vi "Configure Channel.vi"(0 "VISA resource name":refnum<visa-resource-name>, 1 "Enable Channel (T: Enable)":bool=TRUE, 2 "Input Impedance (0: 1M ohm)":u16(ring) items=["1M", "50"], 3 "Bandwidth (0: FULL)":u16(ring) items=["FULL", "500 MHz", "250 MHz", "150 MHz", "20 MHz"], 5 "Channel (0: Channel 1)":u16(ring) format="%#_5f" items=["Channel 1", "Channel 2", "Channel 3", "Channel 4", "Math 1", "Math 2", "Math 3", "Math 4", "Reference 1", "Reference 2", "Reference 3", "Reference 4"], 7 "Vertical Coupling (1: DC)":u16(ring)=1 items=["AC", "DC", "Ground"], 9 "Probe Attenuation (1.0)":dbl=1.0, 11 "error in (no error)":errorcluster, 12 "Vertical Range (10.0 V)":dbl=10.0, 13 "Vertical Offset (0.0 V)":dbl) -> (4 "VISA resource name out":refnum<visa-resource-name>, 15 "error out":errorcluster)   [LabVIEW 2011, in "Tektronix 7000 Series.lvlib"]
doc: "Configures the vertical properties of an oscilloscope for a specified channel. This VI does not configure channel settings for disabled channels."
uses:
  Tektronix 7000 Series.lvlib
panel:
  # "Input Channel Parameters"
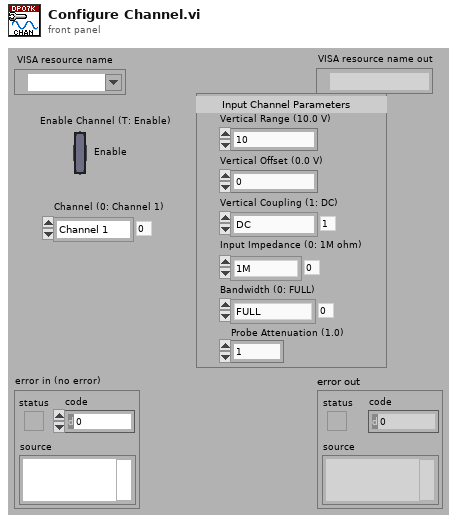
[diagram p1: front panel]
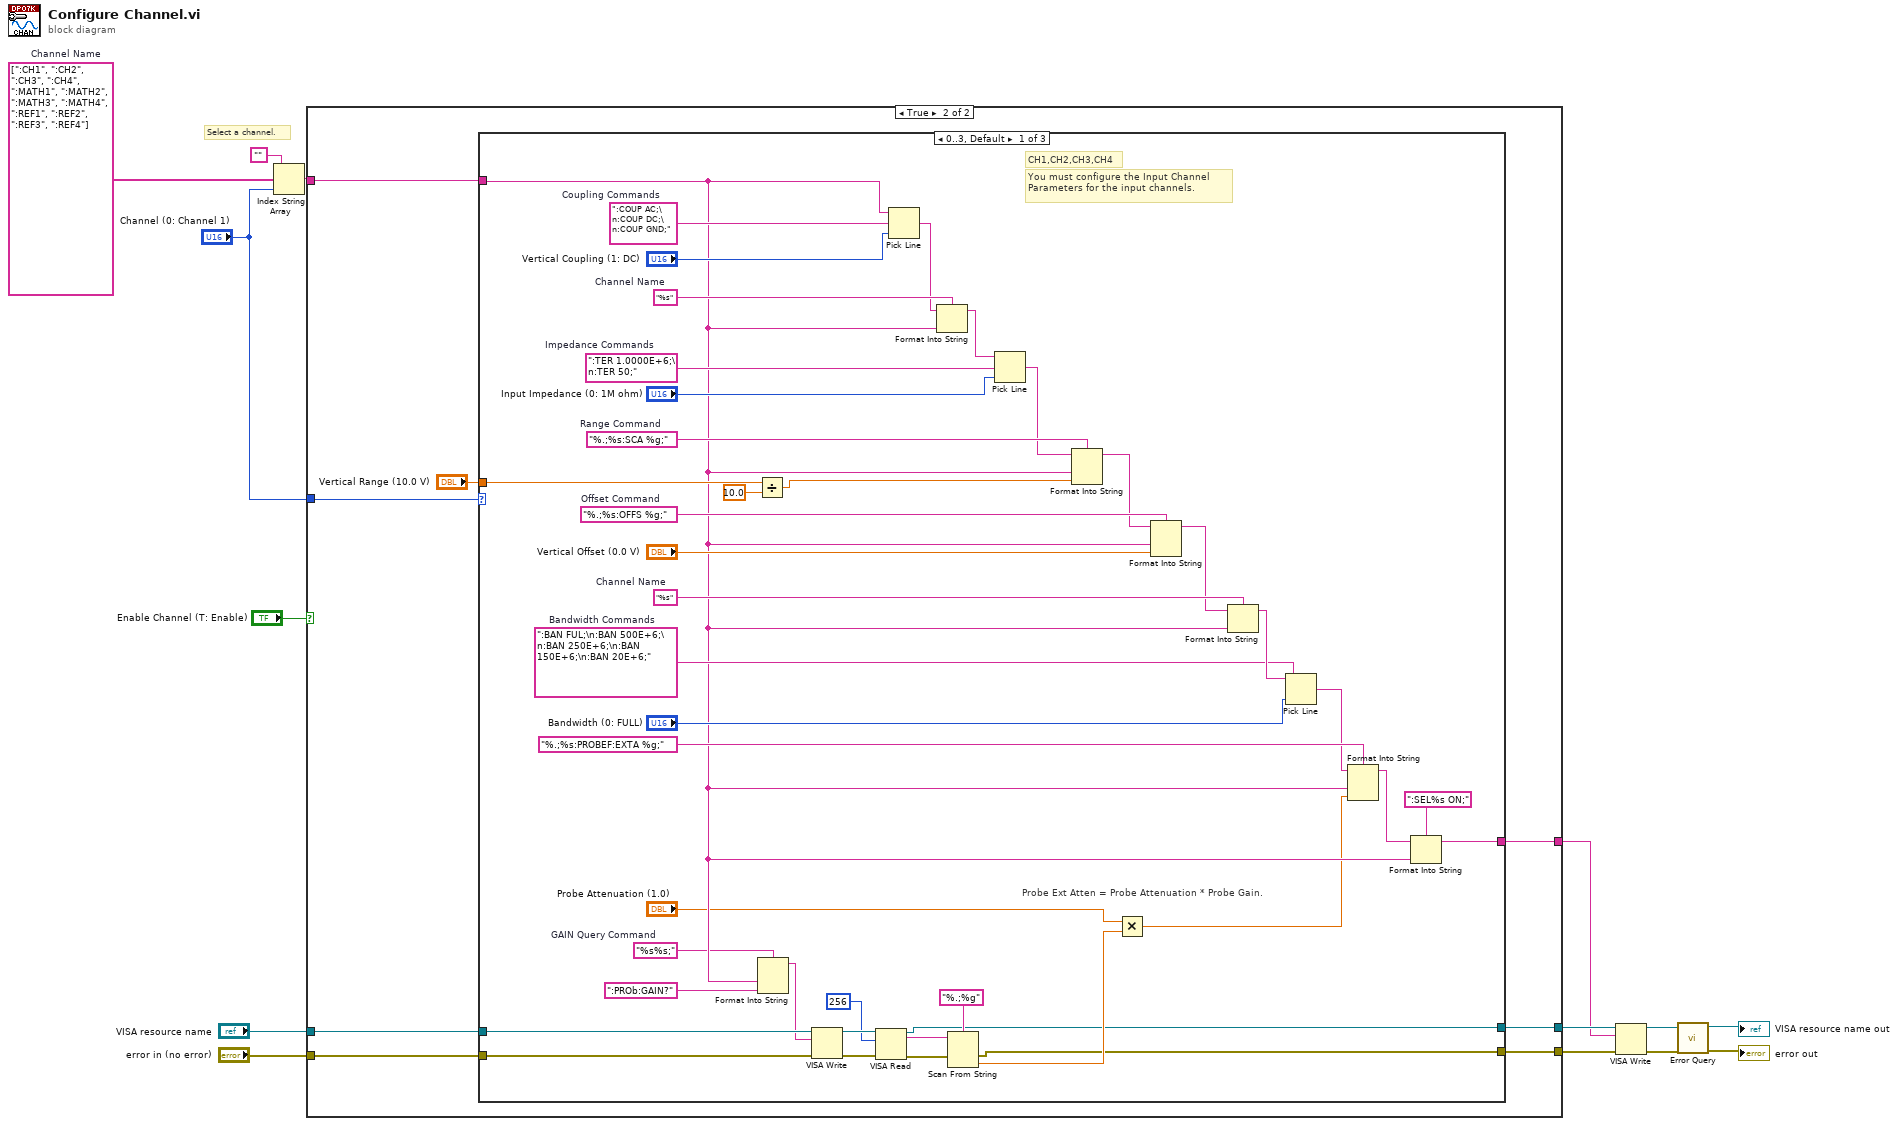
[diagram p0: block diagram]
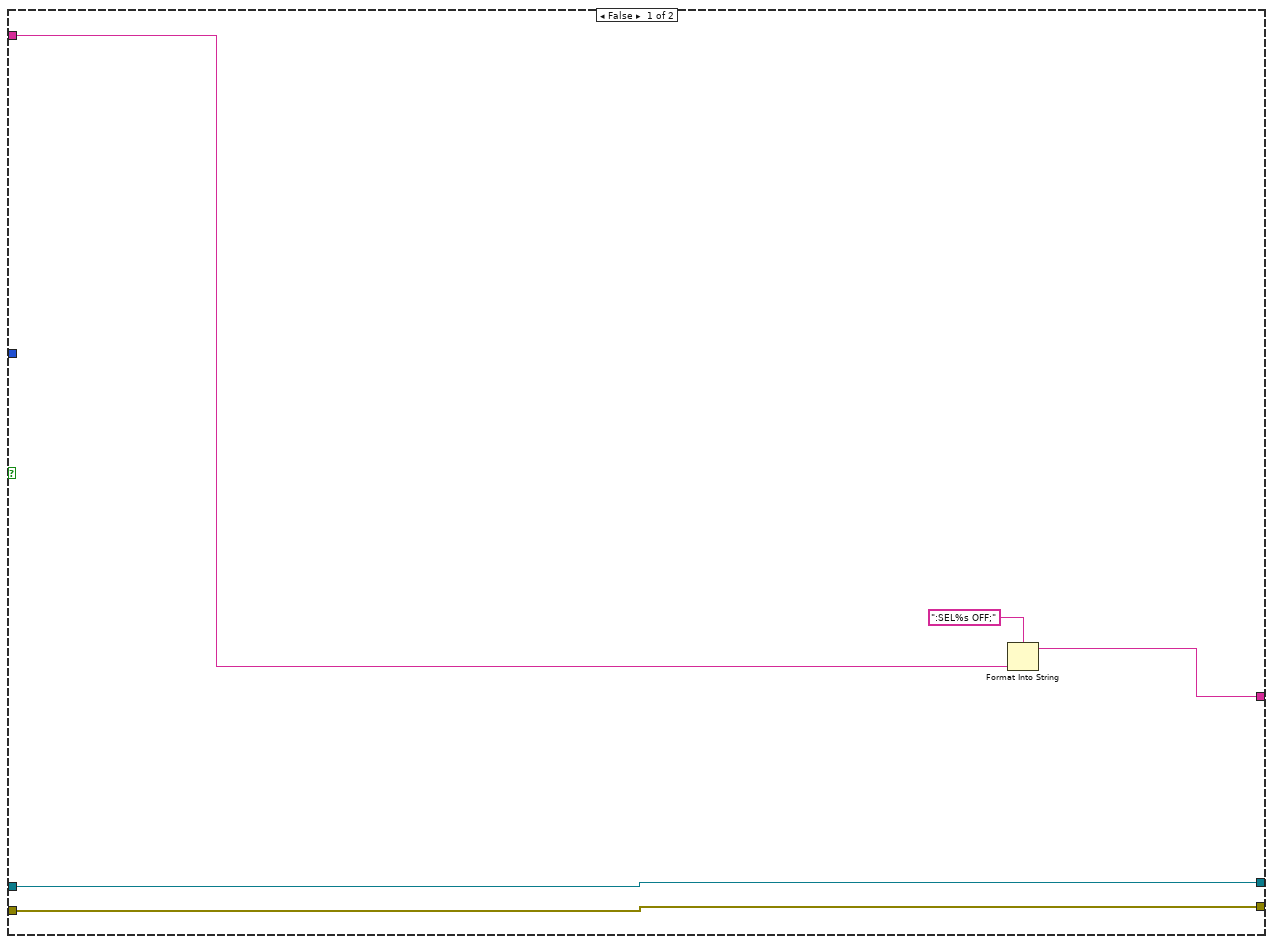
[diagram p2: hidden frame]
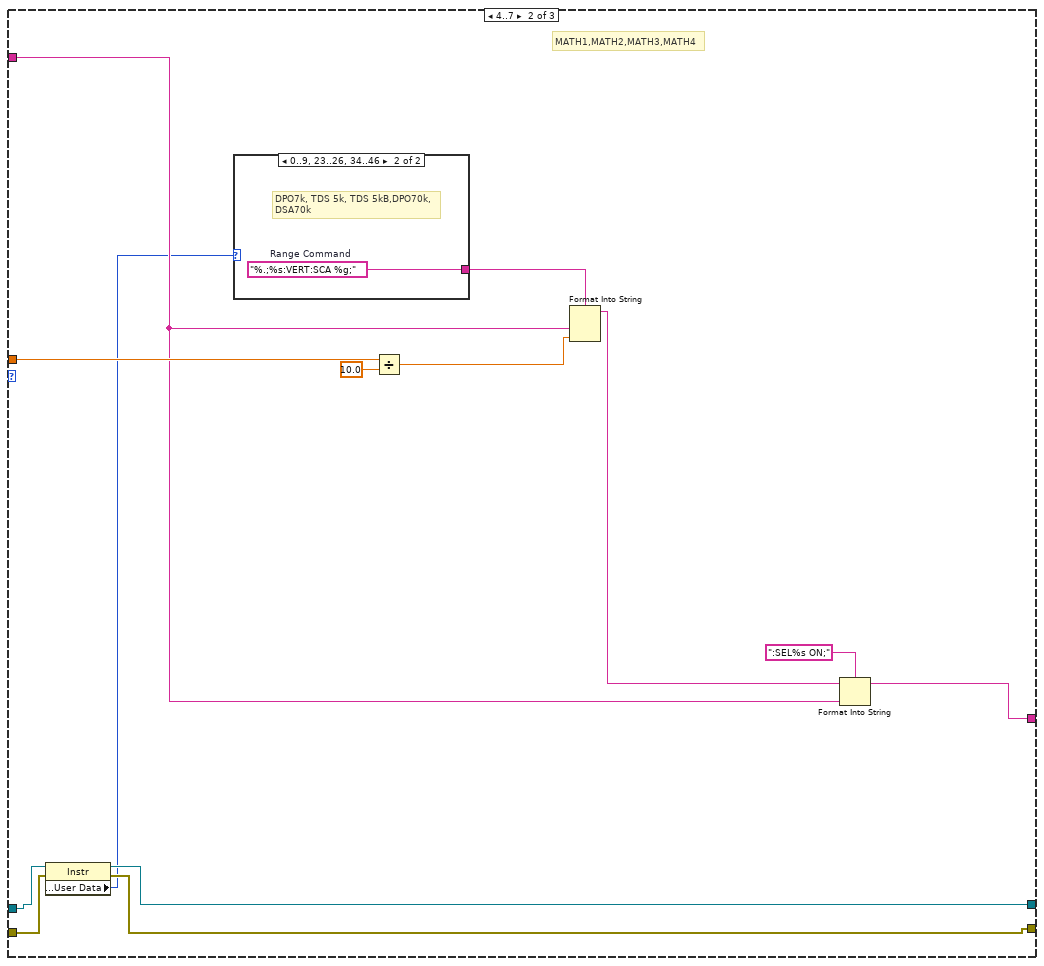
[diagram p3: hidden frame]
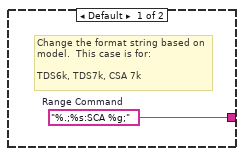
[diagram p4: hidden frame]
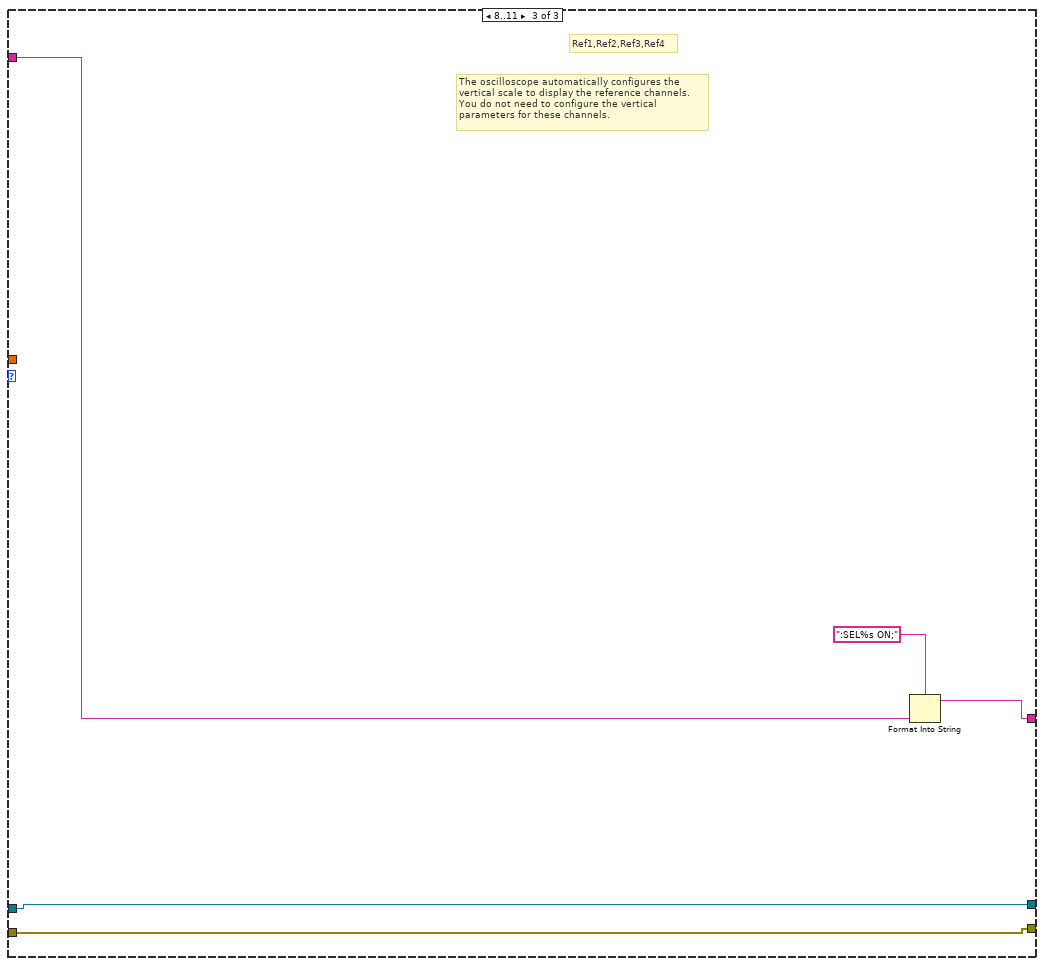
[diagram p5: hidden frame]
diagram:
  w11 = string[] [":CH1", ":CH2", ":CH3", ":CH4", ":MATH1", ":MATH2", ":MATH3", ":MATH4", ":REF1", ":REF2", ":REF3", ":REF4"]  # Channel Name
  # "Select a channel."
  n1 = Index String Array(1:"Channel (0: Channel 1)", 2:w11, 3:"" ("Empty String Constant")) -> (0:w12:string)
  n2 = case shown="True" "Enable Channel (T: Enable)" {
    tunnel: w12 -> [w19 w27]
    tunnel: "Channel (0: Channel 1)" -> [_ w26]
    tunnel: "VISA resource name" -> [w16 w24]
    tunnel: "error in (no error)" -> [w15 w23]
    tunnel: [w16 w22] -> w3
    tunnel: [w15 w21] -> w2
    tunnel: [w17 w20] -> w1
    frame False {
      n3 = Format Into String(format string=":SEL%s OFF;", w19) -> (resulting string=w17:string)  [unwired: 2 in, 1 out]
    }
    frame True {
      n4 = case shown="0..3, Default" w26 {
        tunnel: w27 -> [w42 w77 w88]
        tunnel: "Vertical Range (10.0 V)" -> [w57 w80 _]
        tunnel: w24 -> [w45 w74 w86]
        tunnel: w23 -> [w44 w73 w85]
        tunnel: [w30 w72 w86] -> w22
        tunnel: [w29 w71 w85] -> w21
        tunnel: [w28 w76 w87] -> w20
        frame 0..3, Default {
          w41 = "%s%s;"  # GAIN Query Command
          w48 = "%.;%s:OFFS %g;"  # Offset Command
          w53 = "%s"  # Channel Name
          w54 = ":TER 1.0000E+6;\n:TER 50;"  # Impedance Commands
          w56 = "%.;%s:SCA %g;"  # Range Command
          w65 = ":BAN FUL;\n:BAN 500E+6;\n:BAN 250E+6;\n:BAN 150E+6;\n:BAN 20E+6;"  # Bandwidth Commands
          w67 = "%s"  # Channel Name
          w69 = ":COUP AC;\n:COUP DC;\n:COUP GND;"  # Coupling Commands
          # "CH1,CH2,CH3,CH4"
          # "Probe Ext Atten = Probe Attenuation * Probe Gain."
          # "You must configure the Input Channel\nParameters for the input channels."
          n5 = Divide(x=w57, y=10.0) -> (x/y=w61:dbl)
          n6 = Format Into String(format string=w41, w42, ":PROb:GAIN?" ("write buffer")) -> (resulting string=w40:string)  [unwired: 2 in, 1 out]
          n7 = VISA Write(VISA resource name=w45, write buffer=w40, error in (no error)=w44) -> (VISA resource name out=w39:refnum<visa-resource-name>, error out=w38:errorcluster)  [unwired: 1 out]
          n8 = VISA Read(VISA resource name=w39, byte count=u32 256, error in (no error)=w38) -> (VISA resource name out=w30:refnum<visa-resource-name>, read buffer=w35:string, error out=w36:errorcluster)  [unwired: 1 out]
          n9 = Pick Line(string ("")=w42, multi-line string=w69, line index="Vertical Coupling (1: DC)") -> (output string=w51:string)
          n10 = Format Into String(format string=w53, initial string=w51, w42) -> (resulting string=w52:string)  [unwired: 1 in, 1 out]
          n11 = Scan From String(format string="%.;%g", input string=w35, error in=w36) -> (error out=w29:errorcluster, output 1=w32:dbl)  [unwired: 2 in, 2 out]
          n12 = Pick Line(string ("")=w52, multi-line string=w54, line index="Input Impedance (0: 1M ohm)") -> (output string=w50:string)
          n13 = Format Into String(format string=w56, initial string=w50, w42, w61) -> (resulting string=w47:string)  [unwired: 1 in, 1 out]
          n14 = Multiply(x="Probe Attenuation (1.0)", y=w32) -> (x*y=w31:dbl)
          n15 = Format Into String(format string=w48, initial string=w47, w42, "Vertical Offset (0.0 V)") -> (resulting string=w46:string)  [unwired: 1 in, 1 out]
          n16 = Format Into String(format string=w67, initial string=w46, w42) -> (resulting string=w66:string)  [unwired: 1 in, 1 out]
          n17 = Pick Line(string ("")=w66, multi-line string=w65, line index="Bandwidth (0: FULL)") -> (output string=w59:string)
          n18 = Format Into String(format string="%.;%s:PROBEF:EXTA %g;", initial string=w59, w42, w31) -> (resulting string=w58:string)  [unwired: 1 in, 1 out]
          n19 = Format Into String(format string=":SEL%s ON;", initial string=w58, w42) -> (resulting string=w28:string)  [unwired: 1 in, 1 out]
        }
        frame 4..7 {
          # "MATH1,MATH2,MATH3,MATH4"
          n20 = property class="Instr"(reference=w74, error in=w73) -> (reference out=w72:refnum<visa-resource-name>, error out=w71:errorcluster, "General Settings:User Data"=w70:u32)
          n21 = case shown="0..9, 23..26, 34..46" w70 {
            tunnel: [w83 w84] -> w75
            frame Default {
              w83 = "%.;%s:SCA %g;"  # Range Command
              # "Change the format string based on model.  This case is for:\n\nTDS6k, TDS7k, CSA 7k"
            }
            frame 0..9, 23..26, 34..46 {
              w84 = "%.;%s:VERT:SCA %g;"  # Range Command
              # "DPO7k, TDS 5k, TDS 5kB,DPO70k,\nDSA70k"
            }
          }
          n22 = Divide(x=w80, y=10.0) -> (x/y=w79:dbl)
          n23 = Format Into String(format string=w75, w77, w79) -> (resulting string=w78:string)  [unwired: 2 in, 1 out]
          n24 = Format Into String(format string=":SEL%s ON;", initial string=w78, w77) -> (resulting string=w76:string)  [unwired: 1 in, 1 out]
        }
        frame 8..11 {
          # "Ref1,Ref2,Ref3,Ref4"
          # "The oscilloscope automatically configures the vertical scale to display the reference channels. You do not need to configure the vertical parameters for these channels."
          n25 = Format Into String(format string=":SEL%s ON;", w88) -> (resulting string=w87:string)  [unwired: 2 in, 1 out]
        }
      }
    }
  }
  n26 = VISA Write(VISA resource name=w3, write buffer=w1, error in (no error)=w2) -> (VISA resource name out=w7:refnum<visa-resource-name>, error out=w6:errorcluster)  [unwired: 1 out]
  n27 = call "Error Query.vi"("error in (no error)"=w6, "VISA resource name"=w7) -> ("error out"=→"error out":errorcluster, "VISA resource name out"=→"VISA resource name out":refnum<visa-resource-name>)  [unwired: 6 in, 2 out]
